vi "tm3samp_01_snap.vi"() -> ()   [LabVIEW 2023]
panel:
  out "Image":u16[][](graph)
  out "Error Out":errorcluster
  # "This is just a simple example of how to capture one image from start to finish."
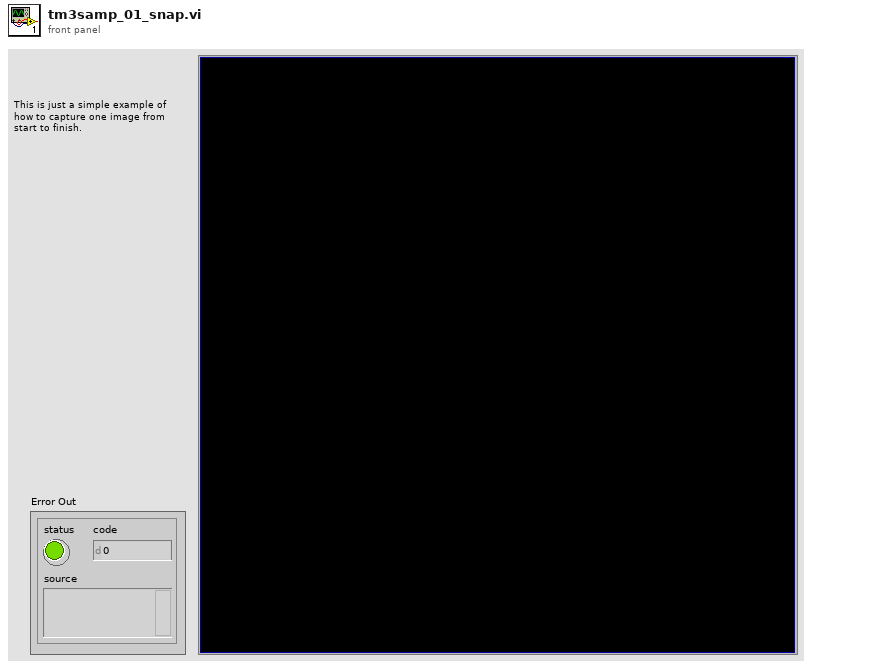
[diagram p1: front panel]
types:
  T1 = cluster{"height":u32, "width":u32, "datatype":u32}
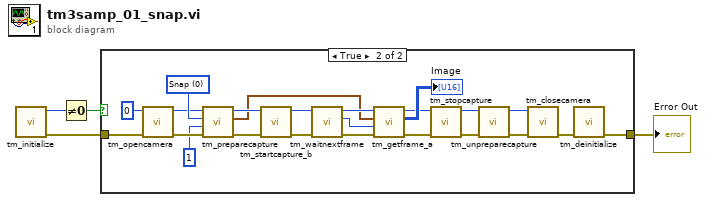
[diagram p0: block diagram]
diagram:
  n1 = call "tm_initialize.vi"() -> ("error out"=w1:errorcluster, "Number Of Cameras"=w2:u32)  [unwired: 8 in, 2 out]
  n2 = Not Equal To 0?(x=w2) -> (x != 0?=w4:bool)
  n3 = case shown="True" w4 {
    tunnel: w1 -> [w5 w28]
    tunnel: [w5 w25] -> w3
    frame False {
    }
    frame True {
      w20 = 0 items=["Snap", "Sequence"] ("Capture mode")
      n4 = call "tm_opencamera.vi"("error in (no error)"=w28, "Camera Index"=u32 0) -> ("error out"=w16:errorcluster, "Handle out"=w17:u32)  [unwired: 7 in, 1 out]
      n5 = call "tm_preparecapture.vi"("error in (no error)"=w16, "Frames"=1, "Capture mode"=w20, "Handle in"=w17) -> ("error out"=w18:errorcluster, "Buffer Info"=w9:T1, "Handle out"=w19:u32)  [unwired: 4 in, 1 out]
      n6 = call "tm_startcapture_b.vi"("error in (no error)"=w18, "Handle in"=w19) -> ("error out"=w13:errorcluster, "Handle out"=w12:u32)  [unwired: 8 in]
      n7 = call "tm_waitnextframe.vi"("error in (no error)"=w13, "Handle in"=w12) -> ("error out"=w11:errorcluster, "Frame Index"=w8:i32, "Handle out"=w10:u32)  [unwired: 6 in, 1 out]
      n8 = call "tm_getframe_a.vi"("error in (no error)"=w11, "Frame Index"=w8, "Buffer Info"=w9, "Handle in"=w10) -> ("error out"=w6:errorcluster, "Data 16"=→"Image":u16[][], "Handle out"=w7:u32)  [unwired: 3 in, 2 out]
      n9 = call "tm_stopcapture.vi"("error in (no error)"=w6, "Handle in"=w7) -> ("error out"=w21:errorcluster, "Handle out"=w22:u32)  [unwired: 8 in]
      n10 = call "tm_unpreparecapture.vi"("error in (no error)"=w21, "Handle in"=w22) -> ("error out"=w24:errorcluster, "Handle out"=w23:u32)  [unwired: 8 in]
      n11 = call "tm_closecamera.vi"("error in (no error)"=w24, "Handle in"=w23) -> ("error out"=w26:errorcluster)  [unwired: 9 in]
      n12 = call "tm_deinitialize.vi"("error in (no error)"=w26) -> ("error out"=w25:errorcluster)  [unwired: 10 in]
    }
  }
  "Error Out" <- w3
